vi "WaitForAcquisitionUpdate.vi"(7 "piint (readout_time_out)":i64, 8 "error in (no error)":errorcluster, 9 "PicamAcquisitionStatus":T1, 10 "PicamAvailableData":T3, 11 "camera handle in":u64) -> (0 "error out":errorcluster, 1 "PicamAcquisitionStatus* status":T1, 2 "PicamAvailableData* (available)":T3, 3 "camera handle out":u64)   [LabVIEW 2019, in "PICam.lvlib"]
uses:
  PICam.lvlib
  types/PicamAvailableData.ctl
  types/PicamAcquisitionStatus.ctl
  types/PicamAcquisitionErrorsMask.ctl
  Picam64.dll
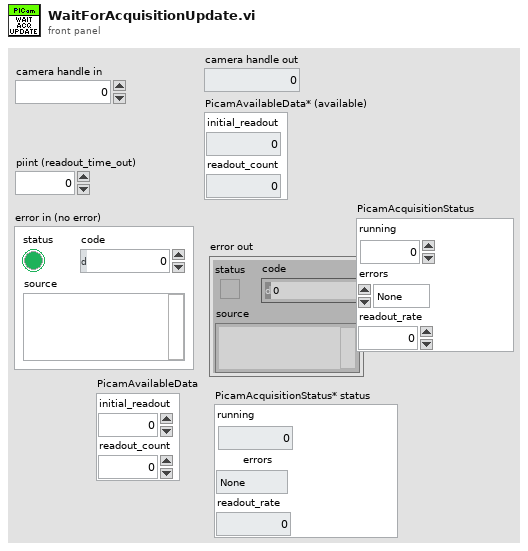
[diagram p1: front panel]
types:
  T1 = typedef "PICam.lvlib/PicamAcquisitionStatus.ctl" = cluster{"running":i32, "errors":T2, "readout_rate":dbl}
  T2 = typedef "PICam.lvlib/PicamAcquisitionErrorsMask.ctl" = enum8{"None", "DataLost", "ConnectionLost", "3", "DataNotArriving", "5", "6", "7", "ShutterOverheated", "9", "10", "11", "12", "13", "14", "15", "CameraFaulted"}
  T3 = typedef "PICam.lvlib/PicamAvailableData.ctl" = cluster{"initial_readout":u64, "readout_count":i64}
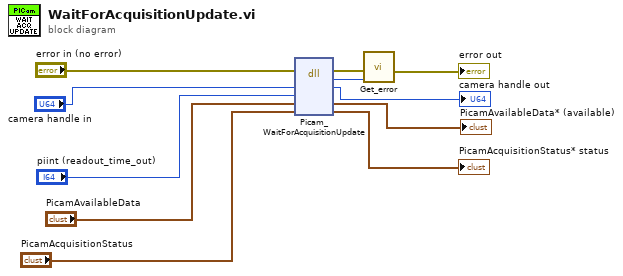
[diagram p0: block diagram]
diagram:
  n1 = dll-call lib="Picam*.*" fn="Picam_WaitForAcquisitionUpdate"(error in="error in (no error)", "PicamHandle (camera)"="camera handle in", "piint (readout_time_out)"="piint (readout_time_out)", "PicamAvailableData* (available)"="PicamAvailableData", "PicamAcquisitionStatus* status"="PicamAcquisitionStatus") -> (error out=w3:errorcluster, "err"=w2:u64, "PicamHandle (camera)"=→"camera handle out":u64, "PicamAvailableData* (available)"=→"PicamAvailableData* (available)":T3, "PicamAcquisitionStatus* status"=→"PicamAcquisitionStatus* status":T1)  [unwired: 3 in, 1 out]
  n2 = call "Get_error.vi"("PICam_Error"=w2, "error in (no error)"=w3) -> ("error out"=→"error out":errorcluster)  [unwired: 9 in]
